vi "Get Type.vi"(11 "I32 1D in":refnum<class "I32 1D.lvclass">) -> (3 "Type":string)   [LabVIEW 2019, in "I32 1D.lvclass"]
uses:
  <vilib>/gpm_packages/@cs/data-type-serializer/source/I32 1D/I32 1D.lvclass
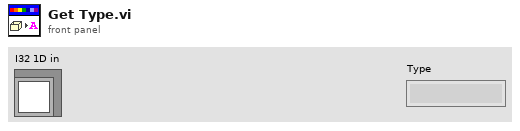
[diagram p1: front panel]
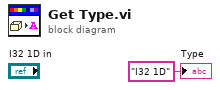
[diagram p0: block diagram]
diagram:
  "Type" <- "I32 1D" ("Type")
